vi "Set Magnet Field.vi"(4 "Mode":T2, 6 "Axis":T1, 8 "error in (no error)":errorcluster, 9 "Target Rate (T/min)":dbl, 10 "Target Field (T)":dbl, 11 "Instrument.VRM in":refnum<class "Instrument.OxfordVRM.lvclass">) -> (0 "error out":errorcluster, 3 "Instrument.VRM out":refnum<class "Instrument.OxfordVRM.lvclass">)   [LabVIEW 2016, in "Instrument.OxfordVRM.lvclass"]
uses:
  Instrument.OxfordVRM.lvclass
  <userlib>/LevyLab/Levylab Instruments/Instrument Types/Cryostat/Typedefs/Magnet Mode--Enum.ctl
  <userlib>/LevyLab/Levylab Instruments/Instrument Types/Cryostat/Typedefs/Magnet Axis--Enum.ctl
  Typedefs/Instrument.VRM.Commands-enum.ctl
  Typedefs/Instrument.VRM.setMagnet-cluster.ctl
  Typedefs/VRM Targets--Cluster.ctl
  <userlib>/LevyLab/Levylab Instruments/Instrument Types/Cryostat/Typedefs/VRM Magnet Axis--Enum.ctl
  <userlib>/LevyLab/Levylab Instruments/Instrument Types/Cryostat/Instrument.Cryostat.lvclass
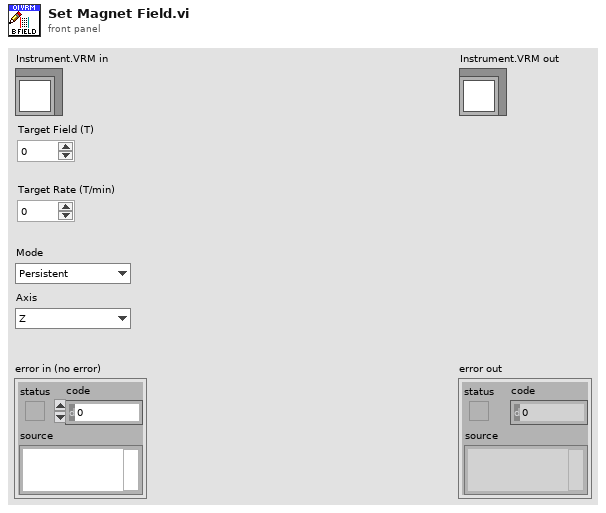
[diagram p1: front panel]
types:
  T1 = typedef "Instrument.Cryostat.lvclass/Magnet Axis--Enum.ctl" = enum16{"Z", "X", "Y"}
  T2 = typedef "Instrument.Cryostat.lvclass/Magnet Mode--Enum.ctl" = enum16{"Persistent", "Driven"}
  T3 = typedef "Instrument.OxfordVRM.lvclass/Instrument.VRM.setMagnet-cluster.ctl" = cluster{"Target":T4}
  T4 = typedef "Instrument.OxfordVRM.lvclass/VRM Targets--Cluster.ctl" = cluster{"Field (T)":dbl, "Field Rate (T/min)":dbl, "Axis":T5}
  T5 = typedef "Instrument.OxfordVRM.lvclass/VRM Magnet Axis--Enum.ctl" = enum16{"Z", "X", "Y", "ALL"}
  T6 = typedef "Instrument.OxfordVRM.lvclass/Instrument.VRM.Commands-enum.ctl" = enum16{"setAction", "setTarget", "setMagnetField", "getStatus", "getTarget", "getMagnetField"}
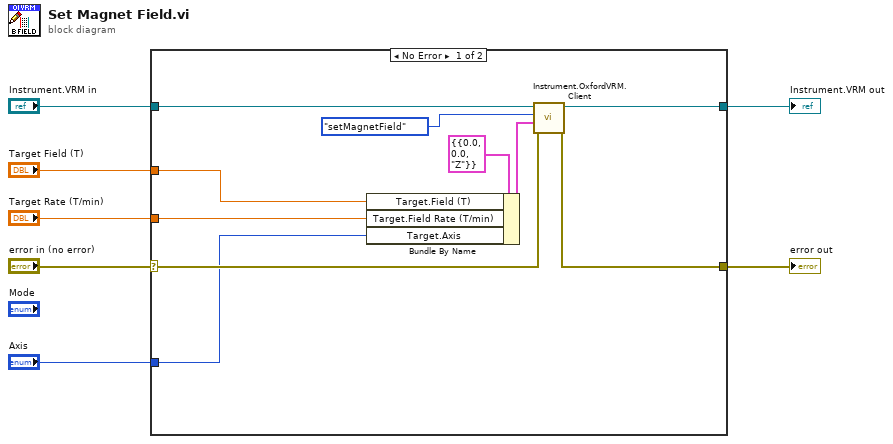
[diagram p0: block diagram]
diagram:
  n1 = case shown="No Error" "error in (no error)" {
    selector: "error in (no error)" -> [w14 w19]
    tunnel: "Target Rate (T/min)" -> [w17 _]
    tunnel: [w13 w19] -> w6
    tunnel: "Target Field (T)" -> [w16 _]
    tunnel: "Instrument.VRM in" -> [w12 w18]
    tunnel: [w15 w18] -> w3
    tunnel: "Axis" -> [w11 _]
    frame No Error {
      n2 = Bundle By Name(cluster=T3 {"Target"={"Field (T)"=0.0, "Field Rate (T/min)"=0.0, "Axis"=enum."Z"}} ("output cluster"), "Target.Field (T)"=w16, "Target.Field Rate (T/min)"=w17, "Target.Axis"=w11) -> (w9:T3)
      n3 = call "Instrument.OxfordVRM.Client.vi"("error in (no error)"=w14, "Data"=w9, "Commands"=Instrument.VRM.Commands-enum."setMagnetField", "Instrument.VRM in"=w12) -> ("error out"=w13:errorcluster, "Instrument.VRM out"=w15:refnum<class "Instrument.OxfordVRM.lvclass">)  [unwired: 5 in, 1 out]
    }
    frame Error {
    }
  }
  "Instrument.VRM out" <- w3
  "error out" <- w6
